vi "Write Child Position.vi"(8 "error in (no error)":errorcluster, 10 "Position":T1, 11 "MDI serialize in":refnum<class "MDI serialize.lvclass">) -> (0 "error out":errorcluster, 3 "MDI serialize out":refnum<class "MDI serialize.lvclass">)   [LabVIEW 2016, in "MDI serialize.lvclass"]
uses:
  MDI serialize.lvclass
  protected/Postion.ctl
  MDI serialize.lvclass/MDI serialize.ctl
  LV MDI.lvclass
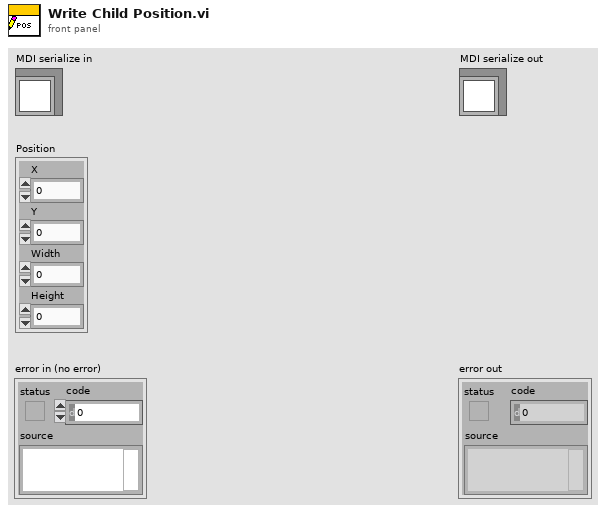
[diagram p1: front panel]
types:
  T1 = typedef "LV MDI.lvclass/Postion.ctl" = cluster{"X":i32, "Y":i32, "Width":i32, "Height":i32}
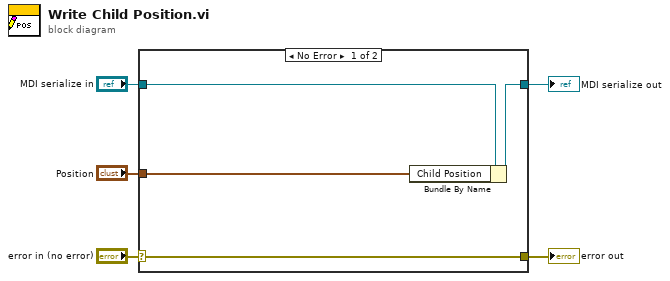
[diagram p0: block diagram]
diagram:
  n1 = case shown="No Error" "error in (no error)" {
    selector: "error in (no error)" -> [w9 w10]
    tunnel: [w9 w10] -> w4
    tunnel: [w7 w11] -> w2
    tunnel: "MDI serialize in" -> [w8 w11]
    tunnel: "Position" -> [w6 _]
    frame No Error {
      n2 = Bundle By Name(cluster=w8, "Child Position"=w6) -> (w7:refnum<class "MDI serialize.lvclass">)
    }
    frame Error {
    }
  }
  "error out" <- w4
  "MDI serialize out" <- w2
